vi "시분초 파일이름.vi"() -> ()   [LabVIEW 2014]
panel:
  out "시간 문자열":string
  out "날짜 문자열":string
  out "날짜/시간 문자열":string
  in  "파일 경로(대화 상자 사용)":path
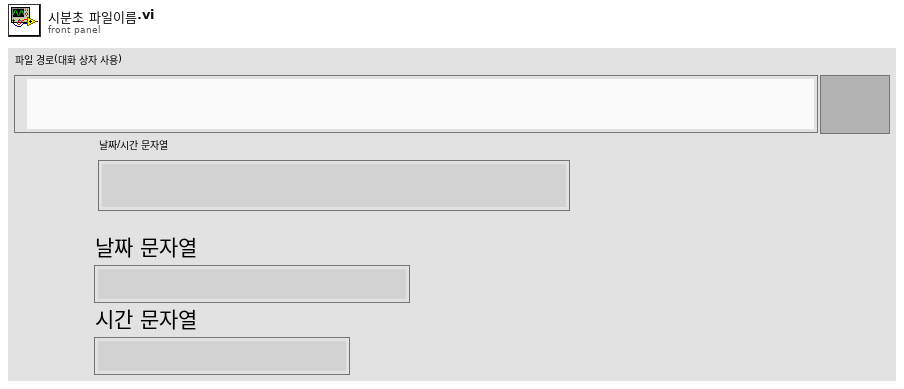
[diagram p1: front panel]
types:
  T1 = enum16{"open", "replace", "create", "open or create", "replace or create", "replace or create with confirmation"}
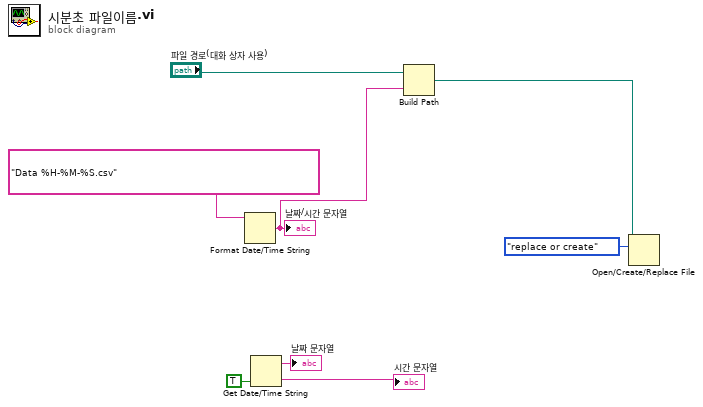
[diagram p0: block diagram]
diagram:
  n1 = Format Date/Time String(time format string (%c)="Data %H-%M-%S.csv" ("시간 포맷 문자열 (%c)")) -> (date/time string=w5:string)  [unwired: 2 in]
  "날짜/시간 문자열" <- w5
  n2 = Get Date/Time String(want seconds? (F)=TRUE ("초 보이기? (거짓)")) -> (date string=→"날짜 문자열":string, time string=→"시간 문자열":string)  [unwired: 2 in]
  n3 = Build Path(base path="파일 경로(대화 상자 사용)", name or relative path=w5) -> (appended path=w4:path)
  n4 = Open/Create/Replace File(file path (use dialog)=w4, operation (0:open)=T1."replace or create" ("동작(0:open)")) -> ()  [unwired: 4 in, 3 out]
